vi "Actor Core.vi"(8 "error in":errorcluster, 11 "cetoni in":refnum<class "cetoni.lvclass">) -> (0 "error out":errorcluster, 3 "Actor out":refnum<class "Actor.lvclass">)   [LabVIEW 2018, in "cetoni.lvlib" / "cetoni.lvclass"]
doc: "(<B>Filename</B>: Actor Framework.lvlib:Actor.lvclass:Actor Core.vi)\n\nReceives messages to the actor, reacts to them, and initiates any error handling that may shut the actor down.\n\nDescendant classes may override this VI to append parallel tasks for the actor to complete while it handles messages. Overrides use the Call Parent Method node."
uses:
  cetoni.lvclass
  <vilib>/ActorFramework/Actor/Actor.lvclass
  cetoni.lvclass/cetoni.ctl
  Resources/GLOBAL/GLOBAL Time-critical.vi
  Device/Device.lvclass
  <userlib>/QmixLib/QmixLib.lvlib
  Program Files/cetoni/QmixSDK/lib/labview/labbCAN_Pump_API/labbCAN_Pump_API.lvlib
panel:
  in  "Stop Button":bool
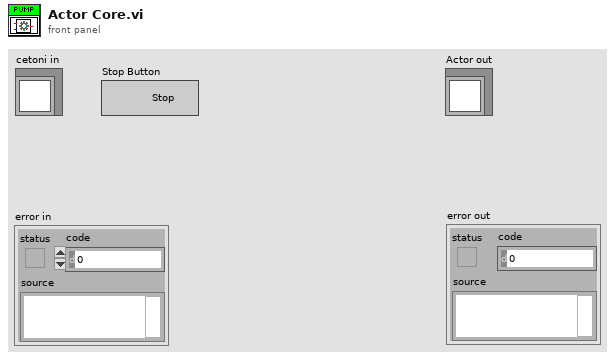
[diagram p1: front panel]
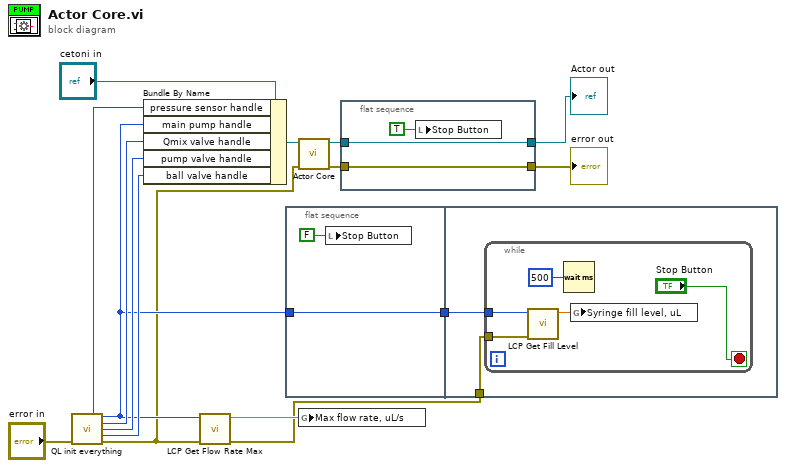
[diagram p0: block diagram]
diagram:
  n1 = call <userlib>:"QL init everything.vi"("error in (no error)"="error in") -> ("pPressureSensor out"=w16:i64, "pMainPump out"=w3:i64, "pQmixValve out"=w15:i64, "pPumpValve out"=w14:i64, "pBallValve out"=w13:i64, "error out"=w1:errorcluster)  [unwired: 9 in]
  n2 = Bundle By Name(cluster="cetoni in", "pressure sensor handle"=w16, "main pump handle"=w3, "Qmix valve handle"=w15, "pump valve handle"=w14, "ball valve handle"=w13) -> (w9:refnum<class "cetoni.lvclass">)
  n3 = call "LCP Get Flow Rate Max.vi"("error in (no error)"=w1, "Pump Handle"=w3) -> ("error out"=w4:errorcluster, "Maximum Flow Rate"=w12:dbl)  [unwired: 8 in]
  n4 = flat-sequence {
    tunnel: w3 -> [w17]
    tunnel: [w17] -> w2
    tunnel: w4 -> [w20]
    tunnel: w2 -> [w19]
    frame #0 {
      n5 = local write "Stop Button"(FALSE ("Stop Button")) -> ()
    }
    frame #1 {
      n6 = while {
        tunnel: w20 -> [w23]
        tunnel: w19 -> [w22]
        stop <- "Stop Button" stop-if-true
        n7 = call "LCP Get Fill Level.vi"("error in (no error)"=w23, "Pump Handle"=w22) -> ("Fill Level"=w21:dbl)  [unwired: 8 in, 1 out]
        n8 = Wait (ms)(milliseconds to wait=u32 500) -> ()  [unwired: 1 out]
        n9 = global write "GLOBAL Time-critical.vi" "Syringe fill level, uL"(w21) -> ()
      }
    }
  }
  n10 = call-parent "Actor Core.vi"("error in"=w1, "Device in"=w9) -> ("error out"=w6:errorcluster, "Actor out"=w8:refnum<class "Actor.lvclass">)  [unwired: 8 in]
  n11 = global write "GLOBAL Time-critical.vi" "Max flow rate, uL/s"(w12) -> ()
  n12 = flat-sequence {
    tunnel: w8 -> [w27]
    tunnel: [w27] -> w7
    tunnel: w6 -> [w26]
    tunnel: [w26] -> w5
    frame #0 {
      n13 = local write "Stop Button"(TRUE ("Stop Button")) -> ()
    }
  }
  "error out" <- w5
  "Actor out" <- w7
